vi "RUSHArmControl.vi"(1 "In Cluster":T3) -> (0 "Out Cluster":T2)   [LabVIEW 2012]
uses:
  <vilib>/Rock Robotics/WPI/Relay/WPI_RelayValue.ctl
panel:
  in  "Setpoint P Gain":dbl=2.0
  in  "Manual P Gain":dbl=2.0
  in  "Vision P Gain":dbl=0.75
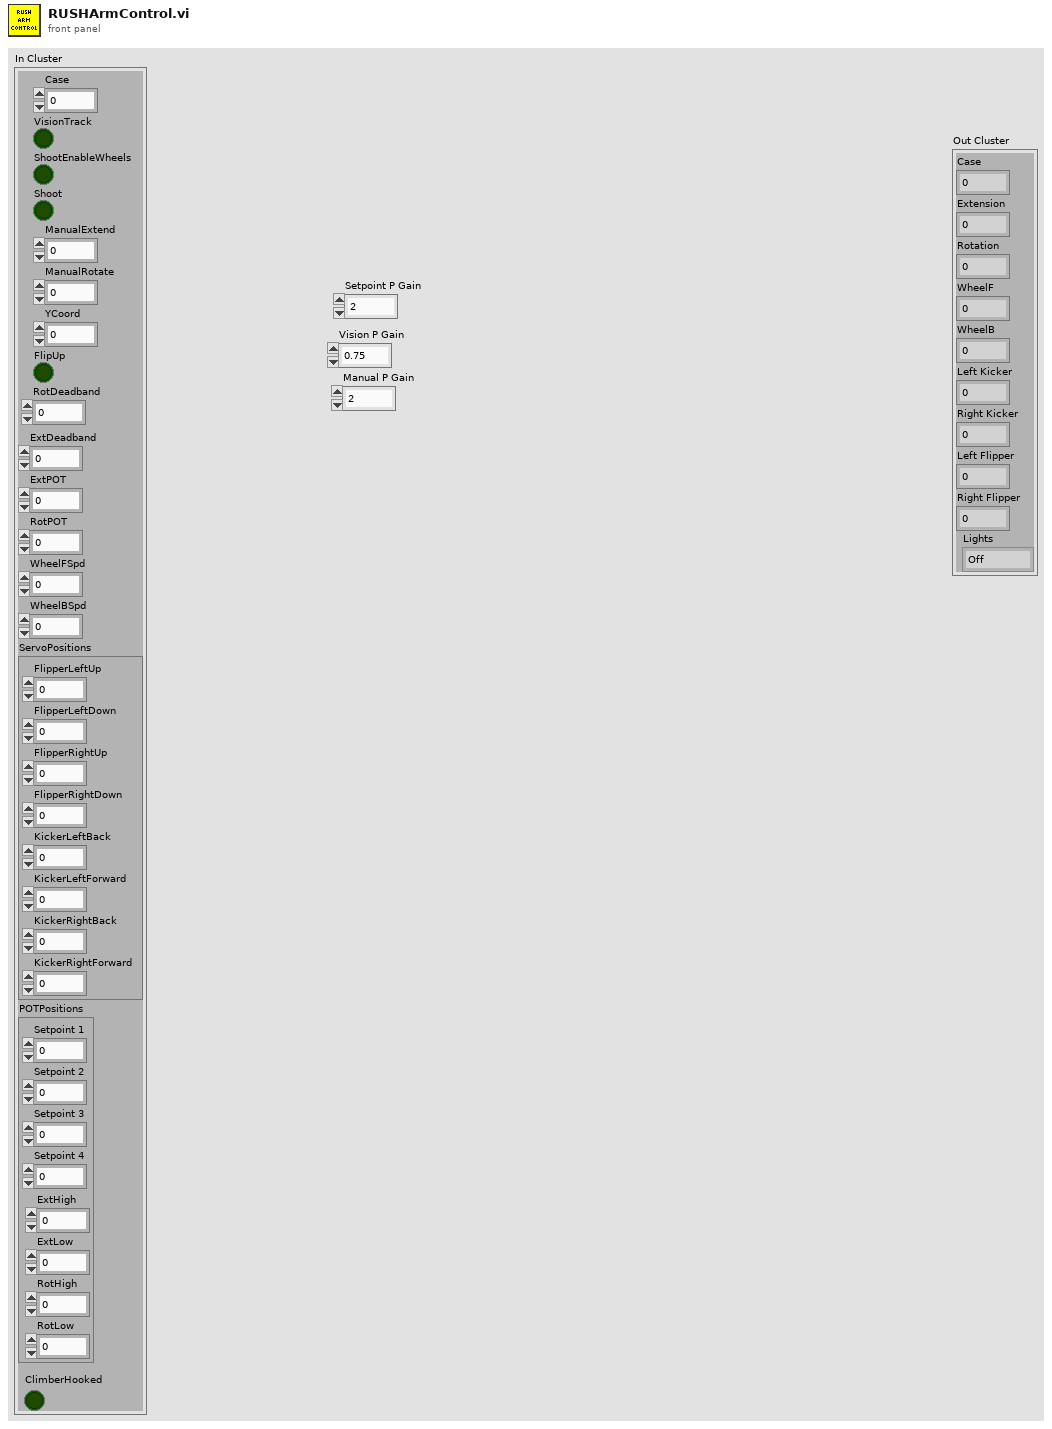
[diagram p1: front panel]
types:
  T1 = typedef "WPI_RelayValue.ctl" = enum16{"Off", "On", "Forward", "Reverse"}
  T2 = cluster{"Case":dbl, "Extension":dbl, "Rotation":dbl, "WheelF":dbl, "WheelB":dbl, "Left Kicker":dbl, "Right Kicker":dbl, "Left Flipper":dbl, "Right Flipper":dbl, "Lights":T1}
  T3 = cluster{"Case":dbl, "VisionTrack":bool, "ShootEnableWheels":bool, "Shoot":bool, "ManualExtend":dbl, "ManualRotate":dbl, "YCoord":dbl, "FlipUp":bool, "RotDeadband":dbl, "ExtDeadband":dbl, "ExtPOT":dbl, "RotPOT":dbl, "WheelFSpd":dbl, "WheelBSpd":dbl, "ServoPositions":cluster{"FlipperLeftUp":dbl, "FlipperLeftDown":dbl, "FlipperRightUp":dbl, "FlipperRightDown":dbl, "KickerLeftBack":dbl, "KickerLeftForward":dbl, "KickerRightBack":dbl, "KickerRightForward":dbl}, "POTPositions":cluster{"Setpoint 1":dbl, "Setpoint 2":dbl, "Setpoint 3":dbl, "Setpoint 4":dbl, "RotLow":dbl, "RotHigh":dbl, "ExtLow":dbl, "ExtHigh":dbl}, "ClimberHooked":bool}
  T4 = cluster{"FlipperLeftUp":dbl, "FlipperLeftDown":dbl, "FlipperRightUp":dbl, "FlipperRightDown":dbl, "KickerLeftBack":dbl, "KickerLeftForward":dbl, "KickerRightBack":dbl, "KickerRightForward":dbl}
  T5 = cluster{"Setpoint 1":dbl, "Setpoint 2":dbl, "Setpoint 3":dbl, "Setpoint 4":dbl, "RotLow":dbl, "RotHigh":dbl, "ExtLow":dbl, "ExtHigh":dbl}
  T6 = cluster{"t":dbl, "y":dbl, "y":dbl, "Output":dbl, "Output":dbl, "KickerLeftBack":dbl, "KickerRightBack":dbl, "FlipperLeftDown":dbl, "FlipperRightDown":dbl, "RelayValue":T1}
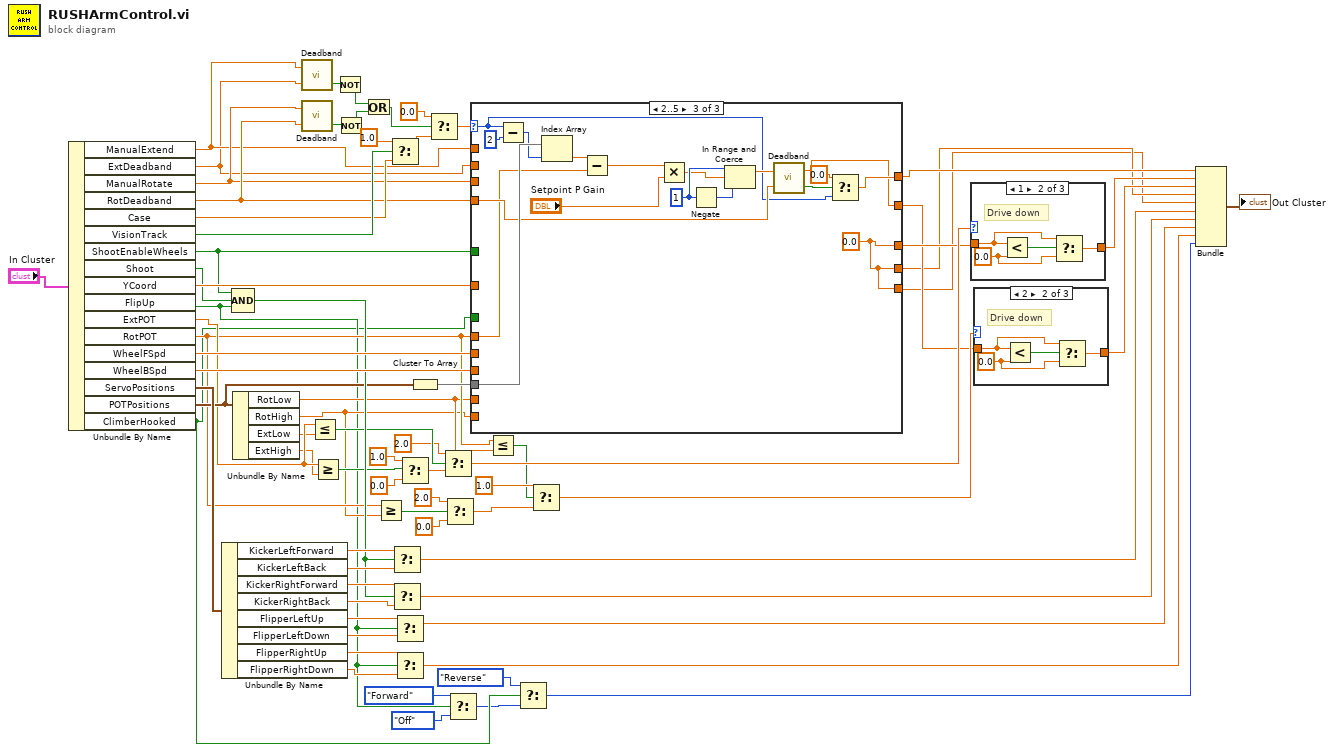
[diagram p0: block diagram]
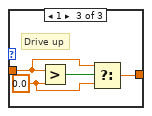
[diagram p3: hidden frame]
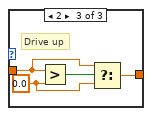
[diagram p5: hidden frame]
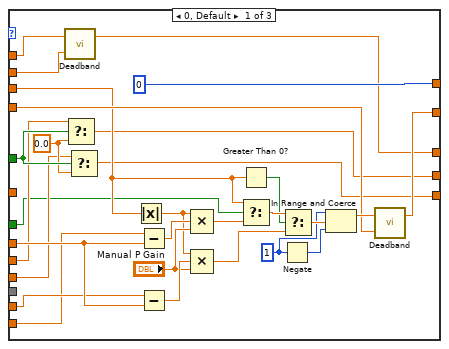
[diagram p6: hidden frame]
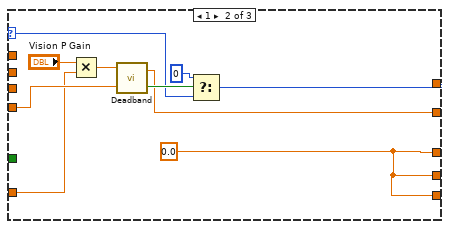
[diagram p7: hidden frame]
diagram:
  n1 = Unbundle By Name("In Cluster") -> ("ManualExtend"=w57:dbl, "ExtDeadband"=w56:dbl, "ManualRotate"=w58:dbl, "RotDeadband"=w60:dbl, "Case"=w61:dbl, "VisionTrack"=w62:bool, "ShootEnableWheels"=w51:bool, "Shoot"=w52:bool, "YCoord"=w59:dbl, "FlipUp"=w7:bool, "ExtPOT"=w34:dbl, "RotPOT"=w22:dbl, "WheelFSpd"=w55:dbl, "WheelBSpd"=w54:dbl, "ServoPositions"=w53:T4, "POTPositions"=w41:T5, "ClimberHooked"=w5:bool)
  n2 = Unbundle By Name(w53) -> ("KickerLeftForward"=w50:dbl, "KickerLeftBack"=w49:dbl, "KickerRightForward"=w48:dbl, "KickerRightBack"=w47:dbl, "FlipperLeftUp"=w45:dbl, "FlipperLeftDown"=w43:dbl, "FlipperRightUp"=w44:dbl, "FlipperRightDown"=w42:dbl)
  n3 = Compound Arithmetic op=AND(w51, w52, w7) -> (w46:bool)
  n4 = Unbundle By Name(w41) -> ("RotLow"=w21:dbl, "RotHigh"=w20:dbl, "ExtLow"=w33:dbl, "ExtHigh"=w32:dbl)
  n5 = call "Deadband.vi"("Deadband"=w56, "Input"=w57) -> ("In Deadband"=w67:bool)  [unwired: 1 out]
  n6 = call "Deadband.vi"("Deadband"=w60, "Input"=w58) -> ("In Deadband"=w66:bool)  [unwired: 1 out]
  n7 = Less Or Equal?(x=w34, y=w33) -> (x <= y?=w35:bool)
  n8 = Greater Or Equal?(x=w34, y=w32) -> (x >= y?=w39:bool)
  n9 = Not(x=w67) -> (.not. x?=w64:bool)
  n10 = Not(x=w66) -> (.not. x?=w65:bool)
  n11 = Or(x=w64, y=w65) -> (x .or. y?=w63:bool)
  n12 = Greater Or Equal?(x=w22, y=w20) -> (x >= y?=w23:bool)
  n13 = Select(t=1.0, s=w62, f=w61) -> (s? t:f=w69:dbl)
  n14 = Select(t=w50, s=w46, f=w49) -> (s? t:f=w12:dbl)
  n15 = Select(t=w48, s=w46, f=w47) -> (s? t:f=w11:dbl)
  n16 = Select(t=w45, s=w7, f=w43) -> (s? t:f=w10:dbl)
  n17 = Select(t=w44, s=w7, f=w42) -> (s? t:f=w9:dbl)
  n18 = Select(t=1.0, s=w39, f=0.0) -> (s? t:f=w36:dbl)
  n19 = Cluster To Array(cluster=w41) -> (array=w40:dbl[])
  n20 = Select(t=0.0, s=w63, f=w69) -> (s? t:f=w72:dbl)
  n21 = Select(t=2.0, s=w35, f=w36) -> (s? t:f=w30:dbl)
  n22 = Select(t=2.0, s=w23, f=0.0) -> (s? t:f=w26:dbl)
  n23 = Select(t=WPI_RelayValue."Forward" ("RelayValue"), s=w7, f=WPI_RelayValue."Off" ("RelayValue")) -> (s? t:f=w4:T1)
  n24 = case shown="2..5" w72 {
    selector: w72 -> [_ w106 w115]
    tunnel: w60 -> [w86 w109 w119]
    tunnel: w59 -> [_ w108 _]
    tunnel: [0 ("t") w104 w114] -> w17
    tunnel: [w84 w103 w113] -> w18
    tunnel: w22 -> [w89 _ w118]
    tunnel: w21 -> [w88 _ _]
    tunnel: w20 -> [w87 _ _]
    tunnel: w58 -> [w85 _ _]
    tunnel: w57 -> [w82 _ _]
    tunnel: w56 -> [w81 _ _]
    tunnel: [w80 w102 w112] -> w29
    tunnel: w51 -> [w79 _ _]
    tunnel: w55 -> [w77 _ _]
    tunnel: w54 -> [w76 _ _]
    tunnel: [w75 w102 w112] -> w14
    tunnel: [w74 w102 w112] -> w13
    tunnel: w40 -> [_ _ w128]
    tunnel: w5 -> [w73 _ _]
    frame 0, Default {
      w78 = 0.0 ("f")
      w91 = 1
      n25 = call "Deadband.vi"("Deadband"=w81, "Input"=w82) -> ("Output"=w80:dbl)  [unwired: 1 out]
      n26 = Select(t=w77, s=w79, f=w78) -> (s? t:f=w75:dbl)
      n27 = Select(t=w76, s=w79, f=w78) -> (s? t:f=w74:dbl)
      n28 = Absolute Value(x=w85) -> (abs(x)=w95:dbl)
      n29 = Subtract(x=w87, y=w89) -> (x-y=w101:dbl)
      n30 = Subtract(x=w88, y=w89) -> (x-y=w100:dbl)
      n31 = Compound Arithmetic op=MULTIPLY(w95, w101, "Manual P Gain") -> (w98:dbl)
      n32 = Compound Arithmetic op=MULTIPLY(w95, w100, "Manual P Gain") -> (w96:dbl)
      n33 = Greater Than 0?(x=w85) -> (x > 0?=w94:bool)
      n34 = Select(t=w85, s=w73, f=w98) -> (s? t:f=w97:dbl)
      n35 = Negate(x=w91) -> (-x=w92:i32)
      n36 = Select(t=w97, s=w94, f=w96) -> (s? t:f=w93:dbl)
      n37 = In Range and Coerce(upper limit=w91, x=w93, lower limit=w92) -> (coerced(x)=w90:dbl)  [unwired: 1 out]
      n38 = call "Deadband.vi"("Deadband"=w86, "Input"=w90) -> ("Output"=w84:dbl)  [unwired: 1 out]
    }
    frame 1 {
      w102 = 0.0 ("Output")
      n39 = Multiply(x="Vision P Gain", y=w108) -> (x*y=w110:dbl)
      n40 = call "Deadband.vi"("Deadband"=w109, "Input"=w110) -> ("In Deadband"=w107:bool, "Output"=w103:dbl)
      n41 = Select(t=0, s=w107, f=w106) -> (s? t:f=w104:i32)
    }
    frame 2..5 {
      w112 = 0.0 ("Output")
      w122 = 1
      n42 = Subtract(x=w115, y=2) -> (x-y=w127:i32)
      n43 = Index Array(array=w128, index=w127) -> (element=w126:dbl)
      n44 = Subtract(x=w126, y=w118) -> (x-y=w125:dbl)
      n45 = Multiply(x=w125, y="Setpoint P Gain") -> (x*y=w121:dbl)
      n46 = Negate(x=w122) -> (-x=w123:i32)
      n47 = In Range and Coerce(upper limit=w122, x=w121, lower limit=w123) -> (coerced(x)=w120:dbl)  [unwired: 1 out]
      n48 = call "Deadband.vi"("Deadband"=w119, "Input"=w120) -> ("In Deadband"=w117:bool, "Output"=w113:dbl)
      n49 = Select(t=0.0, s=w117, f=w115) -> (s? t:f=w114:dbl)
    }
  }
  n50 = Less Or Equal?(x=w22, y=w21) -> (x <= y?=w27:bool)
  n51 = Select(t=WPI_RelayValue."Reverse" ("RelayValue"), s=w5, f=w4) -> (s? t:f=w1:T1)
  n52 = Select(t=1.0, s=w27, f=w26) -> (s? t:f=w19:dbl)
  n53 = case shown="1" w30 {
    tunnel: w29 -> [w130 w132 w136]
    tunnel: [w130 w131 w135] -> w16
    frame 0, Default {
      # "All good"
    }
    frame 1 {
      w133 = 0.0 ("y")
      # "Drive down"
      n54 = Less?(x=w132, y=w133) -> (x < y?=w134:bool)
      n55 = Select(t=w132, s=w134, f=w133) -> (s? t:f=w131:dbl)
    }
    frame 2 {
      w137 = 0.0 ("y")
      # "Drive up"
      n56 = Greater?(x=w136, y=w137) -> (0:w138:bool)
      n57 = Select(t=w136, s=w138, f=w137) -> (s? t:f=w135:dbl)
    }
  }
  n58 = case shown="2" w19 {
    tunnel: w18 -> [w139 w141 w145]
    tunnel: [w139 w140 w144] -> w15
    frame 0, Default {
      # "All good"
    }
    frame 2 {
      w142 = 0.0 ("y")
      # "Drive down"
      n59 = Less?(x=w141, y=w142) -> (x < y?=w143:bool)
      n60 = Select(t=w141, s=w143, f=w142) -> (s? t:f=w140:dbl)
    }
    frame 1 {
      w146 = 0.0 ("y")
      # "Drive up"
      n61 = Greater?(x=w145, y=w146) -> (0:w147:bool)
      n62 = Select(t=w145, s=w147, f=w146) -> (s? t:f=w144:dbl)
    }
  }
  n63 = Bundle("t"=w17, "y"=w16, "y"=w15, "Output"=w14, "Output"=w13, "KickerLeftBack"=w12, "KickerRightBack"=w11, "FlipperLeftDown"=w10, "FlipperRightDown"=w9, "RelayValue"=w1) -> (→"Out Cluster":T6)  [unwired: 1 in]
